vi "Write parameters.vi"(6 "output set time":dbl, 8 "alr value":dbl, 9 "output L":dbl, 10 "output H":dbl=100.0 format="%.2f", 11 "Y_Limiter in":refnum<class "Y_Limiter.lvclass">) -> (3 "Y_Limiter out":refnum<class "Y_Limiter.lvclass">)   [LabVIEW 2019, in "control.lvlib" / "Y_Limiter.lvclass"]
uses:
  Y_Limiter.lvclass
  Y_Limiter.lvclass/Y_Limiter.ctl
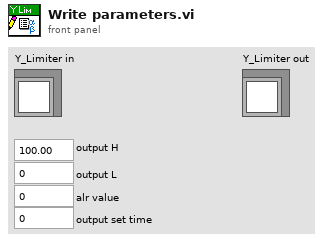
[diagram p1: front panel]
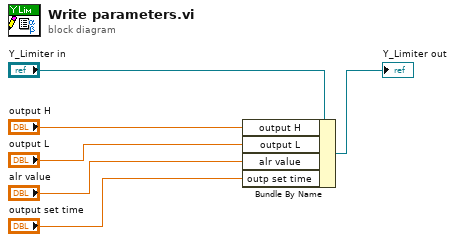
[diagram p0: block diagram]
diagram:
  n1 = Bundle By Name(cluster="Y_Limiter in", "output H"="output H", "output L"="output L", "alr value"="alr value", "outp set time"="output set time") -> (→"Y_Limiter out":refnum<class "Y_Limiter.lvclass">)
